vi "v0.2_dir_serial.vi"(3 "error in (no error)":errorcluster, 4 "Direccion":bool, 5 "VISA COM IN":refnum<visa-resource-name>) -> (0 "error out":errorcluster, 2 "VISA COM OUT":refnum<visa-resource-name>)   [LabVIEW 2011]
doc: "<B>Dirección</B>\n\nCambiar la dirección del Servo Motor de acuerdo al valor de una variable booleana\n\n<B>dir</B> Setear la Dirección"
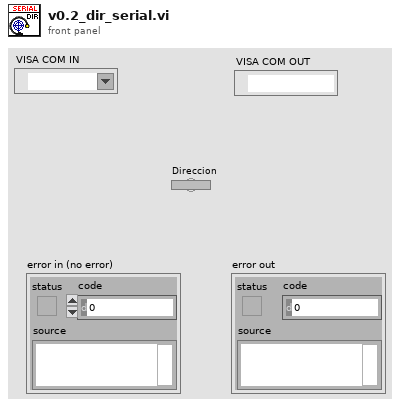
[diagram p1: front panel]
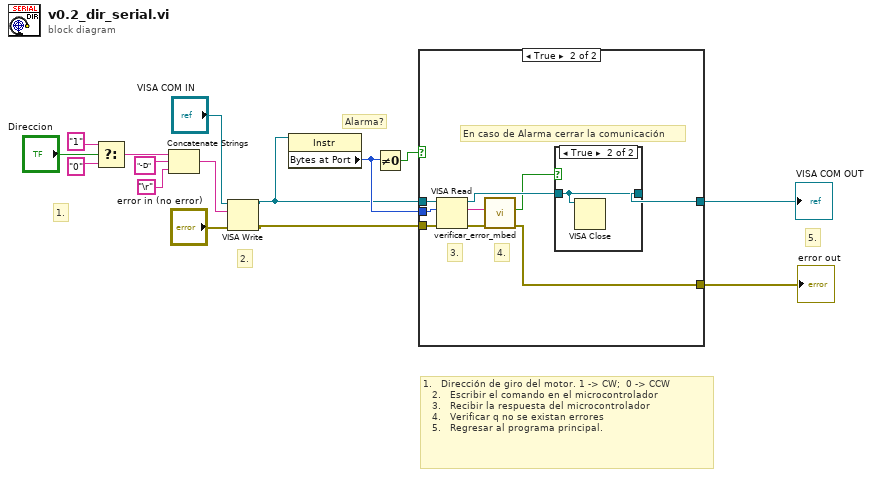
[diagram p0: block diagram]
diagram:
  # "5."
  # "1.   Dirección de giro del motor. 1 -> CW;  0 -> CCW     \n   2.   Escribir el comando en el microcontrolador\n   3.   Recibir la respuesta del microcontrolador\n   4.   Verificar q no se existan errores\n   5.   Regresar al programa principal."
  # "2."
  # "1."
  # "Alarma?"
  n1 = Select(t="1" ("string"), s="Direccion", f="0" ("string")) -> (s? t:f=w8:string)
  n2 = Concatenate Strings(w8, "-D" ("string"), "\r") -> (w13:string)
  n3 = VISA Write(VISA resource name="VISA COM IN", write buffer=w13, error in (no error)="error in (no error)") -> (VISA resource name out=w3:refnum<visa-resource-name>, error out=w4:errorcluster)  [unwired: 1 out]
  n4 = property class="Instr"(reference=w3) -> ("Bytes at Port"=w5:u32)  [unwired: 1 in, 2 out]
  n5 = Not Equal To 0?(x=w5) -> (x != 0?=w6:bool)
  n6 = case shown="True" w6 {
    tunnel: w3 -> [w17 w23]
    tunnel: w4 -> [w16 w22]
    tunnel: w5 -> [_ w21]
    tunnel: [w17 w20] -> w1
    tunnel: [w16 w19] -> w2
    frame False {
    }
    frame True {
      # "4."
      # "3."
      # "En caso de Alarma cerrar la comunicación"
      n7 = VISA Read(VISA resource name=w23, byte count=w21, error in (no error)=w22) -> (VISA resource name out=w24:refnum<visa-resource-name>, read buffer=w25:string, error out=w26:errorcluster)  [unwired: 1 out]
      n8 = call "verificar_error_mbed.vi"("error in (no error)"=w26, "desde_mbed"=w25) -> ("error out"=w19:errorcluster, "error?"=w18:bool)  [unwired: 8 in]
      n9 = case shown="True" w18 {
        tunnel: w24 -> [w27 w28]
        tunnel: [w27 w28] -> w20
        frame False {
        }
        frame True {
          n10 = VISA Close(VISA resource name=w28) -> ()  [unwired: 1 in, 1 out]
        }
      }
    }
  }
  "VISA COM OUT" <- w1
  "error out" <- w2
